vi "Delete Agent Public Key Refnum.vi"(8 "error in (no error)":errorcluster, 11 "agent public key":T1) -> (0 "error out":errorcluster, 3 "libssh2_agent_publickey*":u64)   [LabVIEW 2013, in "libssh2.lvlib"]
doc: "Deletes <B>public key</B> and returns the associated pointer to libssh2_agent_publickey."
uses:
  libssh2.lvlib
  Agent Public Key Refnum.ctl
  Agent Public Key Refnum Data.ctl
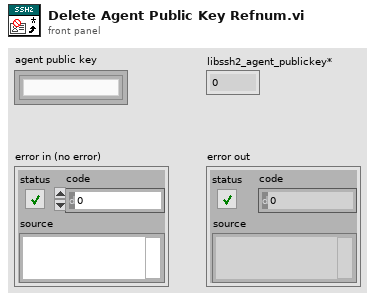
[diagram p1: front panel]
types:
  T1 = typedef "libssh2.lvlib/Agent Public Key Refnum.ctl" = refnum<k1>
  T2 = typedef "libssh2.lvlib/Agent Public Key Refnum Data.ctl" = cluster{"libssh2_agent_publickey*":u64}
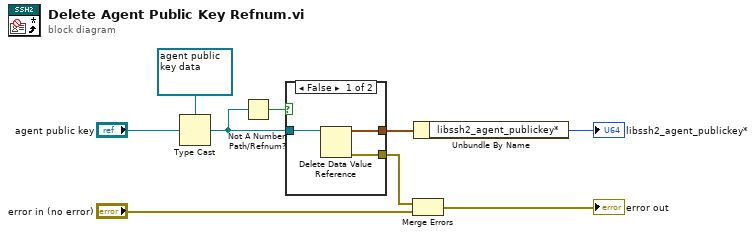
[diagram p0: block diagram]
diagram:
  n1 = Type Cast(type=refnum<data-value> refnum ("data value reference"), x="agent public key") -> (*(type *) &x=w6:refnum<data-value>)
  n2 = Not A Number/Path/Refnum?(number/path/refnum=w6) -> (NaN/Path/Refnum?=w5:bool)
  n3 = case shown="False" w5 {
    tunnel: [w12 _] -> w8
    tunnel: [w11 _] -> w7
    tunnel: w6 -> [w10 _]
    frame False {
      n4 = Delete Data Value Reference(data value reference=w10) -> (data value=w12:T2, error out=w11:errorcluster)  [unwired: 1 in]
    }
    frame True {
    }
  }
  n5 = Merge Errors(w7, "error in (no error)") -> (→"error out":errorcluster)
  n6 = Unbundle By Name(w8) -> ("libssh2_agent_publickey*"=→"libssh2_agent_publickey*":u64)
